vi "closeBothPDs.vi"(8 "error in (no error) 2":errorcluster caption="error in (no error)", 9 "error in (no error)":errorcluster, 10 "instrument handle 2":refnum<visa-resource-name> caption="instrument handle", 11 "instrument handle":refnum<visa-resource-name>) -> (0 "error out 2":errorcluster caption="error out", 3 "error out":errorcluster)   [LabVIEW 2018]
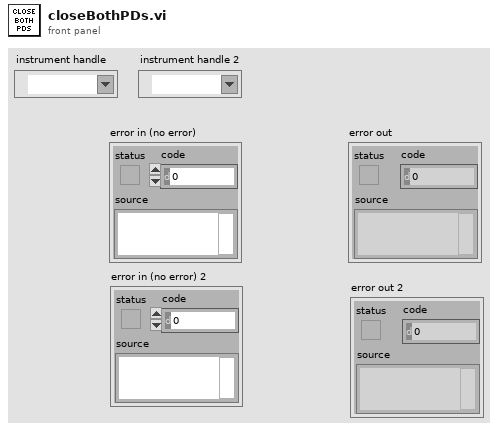
[diagram p1: front panel]
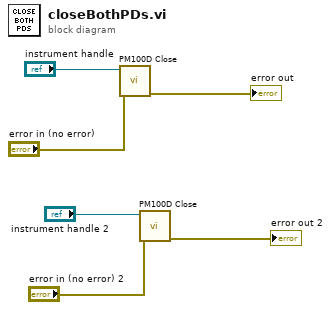
[diagram p0: block diagram]
diagram:
  n1 = call "PM100D Close.vi"("error in (no error)"="error in (no error)", "instrument handle"="instrument handle") -> ("error out"=→"error out":errorcluster)  [unwired: 9 in]
  n2 = call "PM100D Close.vi"("error in (no error)"="error in (no error) 2", "instrument handle"="instrument handle 2") -> ("error out"=→"error out 2":errorcluster)  [unwired: 9 in]
